vi "读取点.vi"(8 "error in (no error)":errorcluster caption="错误输入（无错误）", 11 "点输入":refnum<class "点.lvclass">) -> (0 "error out":errorcluster caption="错误输出", 2 "点":T1, 3 "点输出":refnum<class "点.lvclass">)   [LabVIEW 2011, in "点.lvclass"]
uses:
  <vilib>/Utility/miscctls.llb/LVPointDoubleTypeDef.ctl
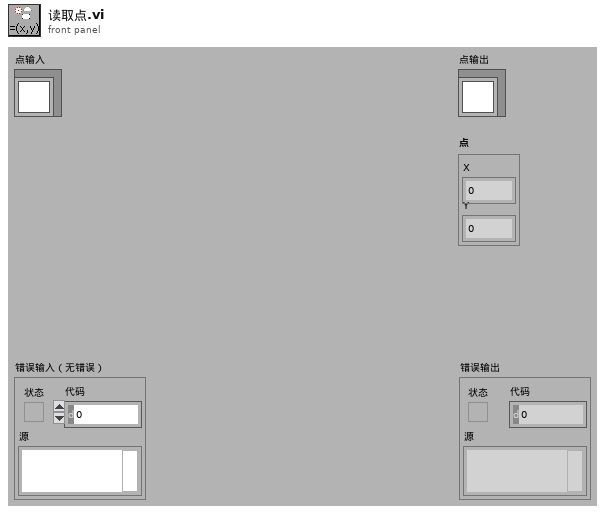
[diagram p1: front panel]
types:
  T1 = typedef "LVPointDoubleTypeDef.ctl" = cluster{"X":dbl, "Y":dbl}
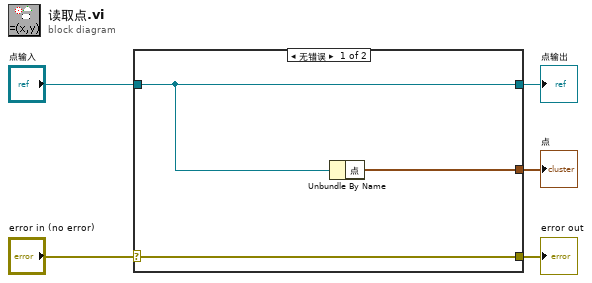
[diagram p0: block diagram]
diagram:
  n1 = case shown="无错误" "error in (no error)" {
    selector: "error in (no error)" -> [w8 w9]
    tunnel: [w8 w9] -> w4
    tunnel: [w7 w10] -> w2
    tunnel: "点输入" -> [w7 w10]
    tunnel: [w6 _] -> w1
    frame No Error {
      n2 = Unbundle By Name(w7) -> ("点"=w6:T1)
    }
    frame Error {
    }
  }
  "error out" <- w4
  "点输出" <- w2
  "点" <- w1
